vi "Launcher.vi"() -> ()   [LabVIEW 2020]
uses:
  UI Controller/UI Controller/UI Controller.lvclass
  C:/Program Files/National Instruments/LabVIEW 2020/vi.lib/ActorFrameworkMVC/View Controller/View Controller/View Controller.lvclass
  C:/Program Files/National Instruments/LabVIEW 2020/vi.lib/ActorFramework/Actor/Actor.lvclass
  UI Controller/UI Controller/UI Controller.lvclass/UI Controller.ctl
  <vilib>/ActorFramework/Message Enqueuer/Message Enqueuer.lvclass/Message Enqueuer.ctl
  UI Controller/UI Controller Messages/Broadcast Close Panel Msg/Broadcast Close Panel Msg.lvclass/Broadcast Close Panel Msg.ctl
  <vilib>/Utility/miscctls.llb/LVPositionTypeDef.ctl
  <vilib>/ActorFrameworkMVC/View Controller/View Controller Messages/Insert Subpanel Msg/Insert Subpanel Msg.lvclass/Insert Subpanel Msg.ctl
  <vilib>/ActorFrameworkMVC/View Controller/View Controller Messages/Move Subpanel Msg/Move Subpanel Msg.lvclass/Move Subpanel Msg.ctl
  UI Controller/UI Controller Messages/Hide Subpanels Msg/Hide Subpanels Msg.lvclass/Hide Subpanels Msg.ctl
  <vilib>/ActorFramework/Message Enqueuer/Enqueue.vi
  UI Controller/UI Controller Messages/Register Data Msg/Register Data Msg.lvclass
  C:/Program Files/National Instruments/LabVIEW 2020/vi.lib/ActorFramework/Message/Message.lvclass
  UI Controller/UI Controller Messages/Broadcast Close Panel Msg/Broadcast Close Panel Msg.lvclass
  <vilib>/ActorFrameworkMVC/View Controller/View Controller Messages/Insert Subpanel Msg/Insert Subpanel Msg.lvclass
  <vilib>/ActorFrameworkMVC/View Controller/View Controller Messages/Move Subpanel Msg/Move Subpanel Msg.lvclass
  UI Controller/UI Controller Messages/Hide Subpanels Msg/Hide Subpanels Msg.lvclass
  UI Controller/UI Controller Messages/Update Occupied Area Msg/Update Occupied Area Msg.lvclass
  <vilib>/ActorFramework/Stop Msg/Stop Msg.lvclass
  <vilib>/ActorFramework/Message Priority Queue/Priority Enqueue.vi
  <vilib>/ActorFrameworkMVC/View Controller/View Controller/View Controller.lvclass
  <vilib>/ActorFramework/Actor/Actor.lvclass
  UI Controller/UI Controller.lvlib
panel:
  in  "Menu Button":bool
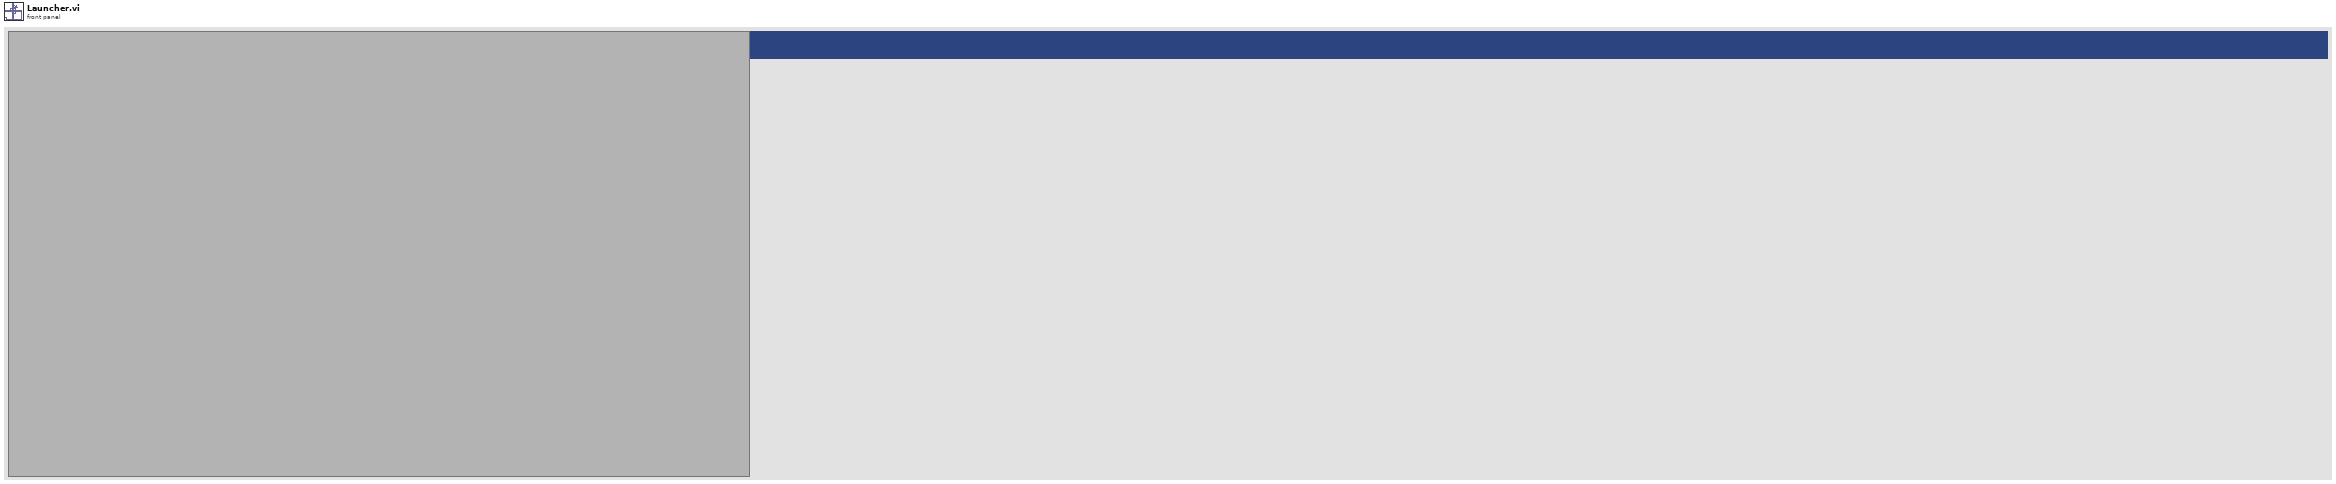
[diagram p1: front panel]
types:
  T1 = typedef "LVBoundsTypeDef.ctl" = cluster{"Width":u32, "Height":u32}
  T2 = typedef "LVPositionTypeDef.ctl" = cluster{"Left":i32, "Top":i32}
  T3 = typedef "LVPoint32TypeDef.ctl" = cluster{"Horizontal":i32, "Vertical":i32}
  T4 = typedef "LVRectTypeDef.ctl" = cluster{"Left":i16, "Top":i16, "Right":i16, "Bottom":i16}
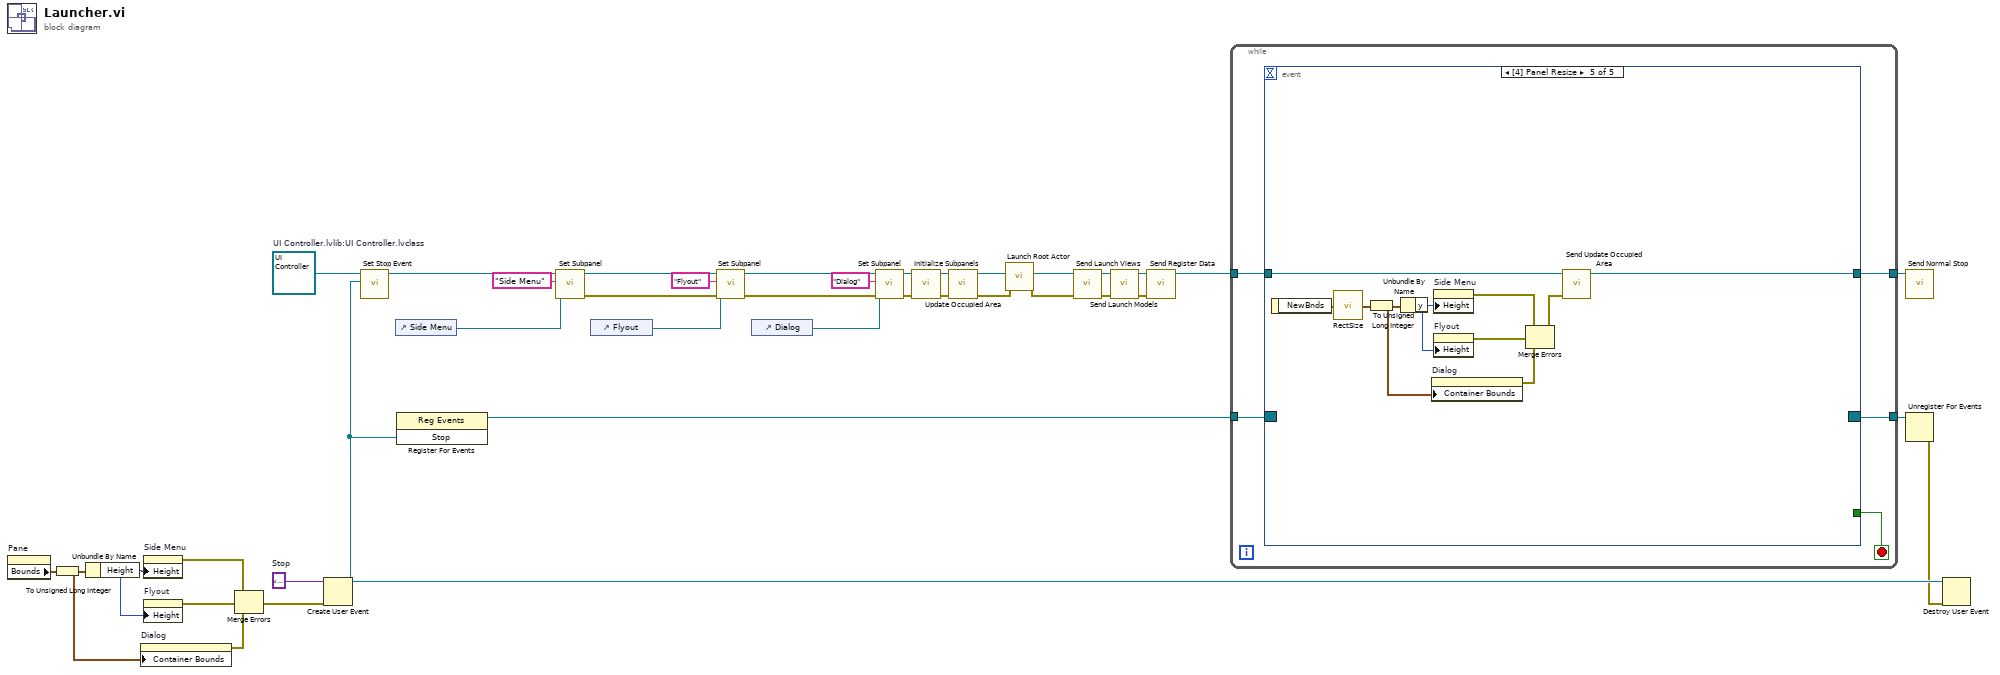
[diagram p0: block diagram]
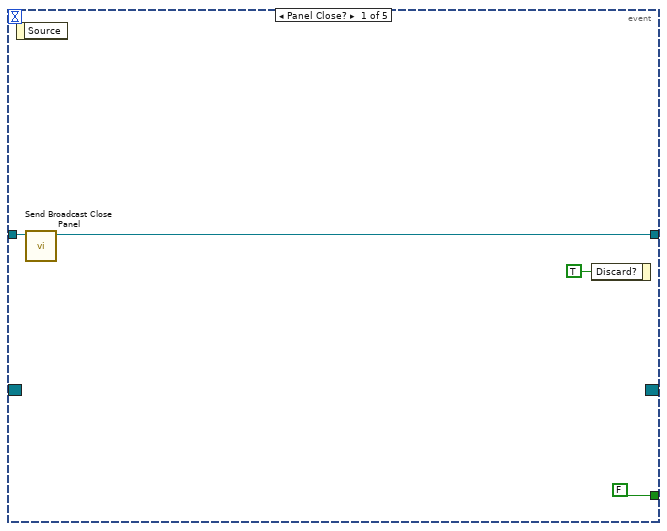
[diagram p2: hidden frame]
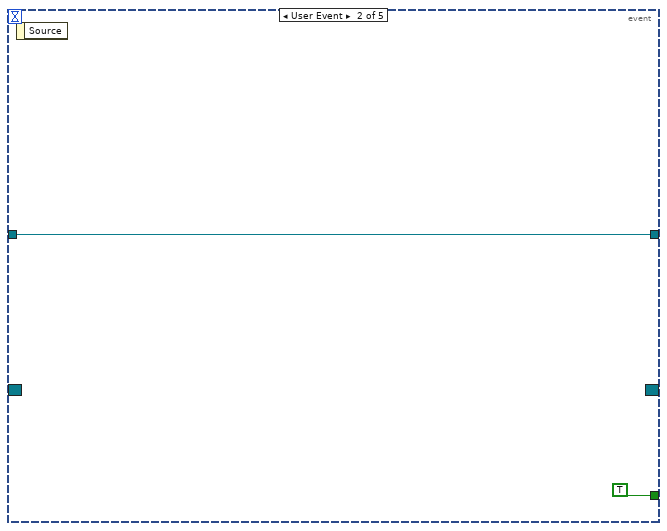
[diagram p3: hidden frame]
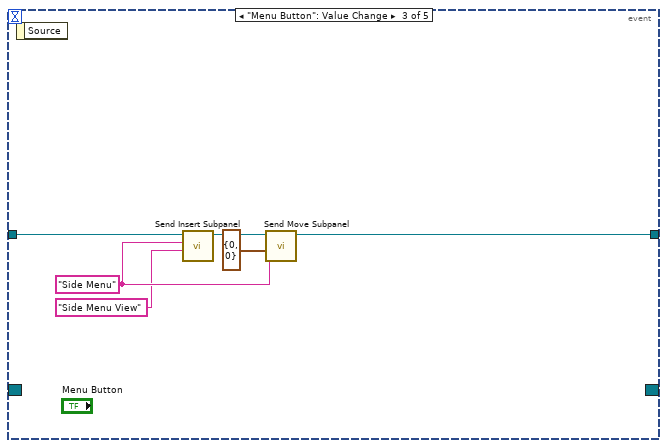
[diagram p4: hidden frame]
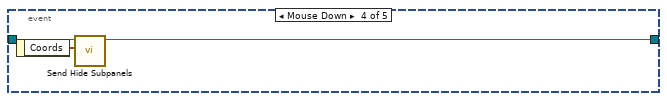
[diagram p5: hidden frame]
diagram:
  w21 = variant  # Stop
  w34 = refnum<class "UI Controller.lvclass"> refnum  # UI Controller.lvlib:UI Controller.lvclass
  n1 = property on="Pane" class="Pane"() -> ("Bounds"=w6:T1)  [unwired: 2 in, 2 out]
  n2 = To Unsigned Long Integer(number=w6) -> (unsigned 32bit integer=w9:T1)
  n3 = Unbundle By Name(w9) -> ("Height"=w11:u32)
  n4 = property on="Dialog" class="SubPnl"("Container Bounds"=w9) -> (error out=w8:errorcluster)  [unwired: 2 in, 1 out]
  n5 = property on="Side Menu" class="SubPnl"("Height"=w11) -> (error out=w10:errorcluster)  [unwired: 2 in, 1 out]
  n6 = property on="Flyout" class="SubPnl"("Height"=w11) -> (error out=w7:errorcluster)  [unwired: 2 in, 1 out]
  n7 = Merge Errors(w10, w7, w8) -> (w5:errorcluster)
  n8 = Create User Event(user event datatype=w21, error in=w5) -> (user event=w17:refnum<user-event>)  [unwired: 1 out]
  n9 = call "Set Stop Event.vi"("Stop Event"=w17, "UI Controller in"=w34) -> ("UI Controller out"=w20:refnum<class "UI Controller.lvclass">)  [unwired: 9 in]
  n10 = control-ref of="Side Menu"() -> (w30:refnum<vi>)
  n11 = register-events(w17) -> (reference out=w19:refnum<event-registration>)  [unwired: 2 in, 1 out]
  n12 = call <vilib>:"Set Subpanel.vi"("Subpanel Reference"=w30, "Subpanel Name"="Side Menu", "View Controller in"=w20) -> ("error out"=w37:errorcluster, "View Controller out"=w38:refnum<class "UI Controller.lvclass">)  [unwired: 7 in]
  n13 = control-ref of="Flyout"() -> (w29:refnum<vi>)
  n14 = call <vilib>:"Set Subpanel.vi"("error in (no error)"=w37, "Subpanel Reference"=w29, "Subpanel Name"="Flyout", "View Controller in"=w38) -> ("error out"=w35:errorcluster, "View Controller out"=w36:refnum<class "UI Controller.lvclass">)  [unwired: 6 in]
  n15 = control-ref of="Dialog"() -> (w28:refnum<vi>)
  n16 = call <vilib>:"Set Subpanel.vi"("error in (no error)"=w35, "Subpanel Reference"=w28, "Subpanel Name"="Dialog", "View Controller in"=w36) -> ("error out"=w23:errorcluster, "View Controller out"=w24:refnum<class "UI Controller.lvclass">)  [unwired: 6 in]
  n17 = call "Initialize Subpanels.vi"("error in (no error)"=w23, "UI Controller in"=w24) -> ("error out"=w22:errorcluster, "UI Controller out"=w2:refnum<class "UI Controller.lvclass">)  [unwired: 8 in]
  n18 = call "Update Occupied Area.vi"("error in (no error)"=w22, "UI Controller in"=w2) -> ("error out"=w3:errorcluster, "UI Controller out"=w1:refnum<class "UI Controller.lvclass">)  [unwired: 8 in]
  n19 = call <vilib>:"Launch Root Actor.vi"("error in (no error)"=w3, "Actor"=w1) -> ("error out"=w14:errorcluster, "Actor's Enqueuer"=w27:refnum<class "Message Enqueuer.lvclass">)  [unwired: 8 in]
  n20 = call "Send Launch Views.vi"("error in (no error)"=w14, "Message Enqueuer in"=w27) -> ("error out"=w16:errorcluster, "Message Enqueuer out"=w25:refnum<class "Message Enqueuer.lvclass">)  [unwired: 8 in]
  n21 = call "Send Launch Models.vi"("error in (no error)"=w16, "Message Enqueuer in"=w25) -> ("error out"=w13:errorcluster, "Message Enqueuer out"=w15:refnum<class "Message Enqueuer.lvclass">)  [unwired: 8 in]
  n22 = call "Send Register Data.vi"("error in (no error)"=w13, "Message Enqueuer"=w15) -> ("Message Enqueuer out"=w4:refnum<class "Message Enqueuer.lvclass">)  [unwired: 8 in, 1 out]
  n23 = while {
    tunnel: w4 -> [w43]
    tunnel: [w42] -> w26
    tunnel: w19 -> [w40]
    tunnel: [w39] -> w18
    stop <- w41 stop-if-true
    n24 = event shown="[4] Panel Resize" {
      selector: w40 -> [_ _ _ _ _]
      dyn-events: [_ _ _ _ _] -> w39
      timeout: _ -> [_ _ _ _ _]
      tunnel: w43 -> [w45 w48 w55 w58 w68]
      tunnel: [w44 w48 w53 w57 w66] -> w42
      tunnel: [FALSE TRUE _ _ _] -> w41
      event Panel Close? {
        n25 = event-data() -> ()  [unwired: 1 in, 1 out]
        n26 = call "Send Broadcast Close Panel.vi"("Message Enqueuer"=w45) -> ("Message Enqueuer out"=w44:refnum<class "Message Enqueuer.lvclass">)  [unwired: 9 in, 1 out]
        n27 = event-data("Discard?"=TRUE) -> ()  [unwired: 1 in, 1 out]
      }
      event User Event {
        n28 = event-data() -> ()  [unwired: 1 in, 1 out]
      }
      event "Menu Button": Value Change {
        w52 = "Side Menu" ("Subpanel Name")
        n29 = event-data() -> ()  [unwired: 1 in, 1 out]
        n30 = call <vilib>:"Send Insert Subpanel.vi"("View Name"="Side Menu View", "Subpanel Name"=w52, "Message Enqueuer"=w55) -> ("Message Enqueuer out"=w54:refnum<class "Message Enqueuer.lvclass">)  [unwired: 7 in, 1 out]
        n31 = call <vilib>:"Send Move Subpanel.vi"("Position"=T2 {"Left"=0, "Top"=0}, "Subpanel Name"=w52, "Message Enqueuer"=w54) -> ("Message Enqueuer out"=w53:refnum<class "Message Enqueuer.lvclass">)  [unwired: 7 in, 1 out]
      }
      event Mouse Down {
        n32 = event-data() -> ("Coords"=w56:T3)  [unwired: 1 in]
        n33 = call "Send Hide Subpanels.vi"("Mouse Down Position"=w56, "Message Enqueuer"=w58) -> ("Message Enqueuer out"=w57:refnum<class "Message Enqueuer.lvclass">)  [unwired: 8 in, 1 out]
      }
      event Panel Resize {
        n34 = event-data() -> ("NewBnds"=w62:T4)  [unwired: 1 in]
        n35 = call <vilib>:"RectSize.vi"("rect"=w62) -> ("point"=w67:cluster{"x":i16, "y":i16})
        n36 = To Unsigned Long Integer(number=w67) -> (unsigned 32bit integer=w61:cluster{"x":u32, "y":u32})
        n37 = Unbundle By Name(w61) -> ("y"=w59:u32)
        n38 = property on="Dialog" class="SubPnl"("Container Bounds"=w61) -> (error out=w64:errorcluster)  [unwired: 2 in, 1 out]
        n39 = property on="Side Menu" class="SubPnl"("Height"=w59) -> (error out=w60:errorcluster)  [unwired: 2 in, 1 out]
        n40 = property on="Flyout" class="SubPnl"("Height"=w59) -> (error out=w65:errorcluster)  [unwired: 2 in, 1 out]
        n41 = Merge Errors(w60, w65, w64) -> (w63:errorcluster)
        n42 = call "Send Update Occupied Area.vi"("error in (no error)"=w63, "Message Enqueuer"=w68) -> ("Message Enqueuer out"=w66:refnum<class "Message Enqueuer.lvclass">)  [unwired: 8 in, 1 out]
      }
    }
  }
  n43 = call <vilib>:"Send Normal Stop.vi"("Message Enqueuer"=w26) -> ()  [unwired: 10 in, 1 out]
  n44 = Unregister For Events(event registration refnum=w18) -> (error out=w12:errorcluster)  [unwired: 1 in]
  n45 = Destroy User Event(user event=w17, error in=w12) -> ()  [unwired: 1 out]
